vi "state_machine.vi"() -> ()   [LabVIEW 2023]
uses:
  typedefs/state_machine_types.ctl
panel:
  out "State":string
  in  "Up State":bool
  in  "Down State":bool
  in  "Stop Button":bool
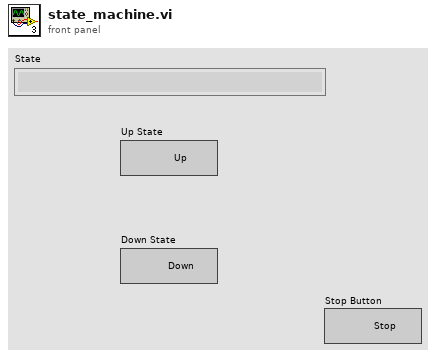
[diagram p1: front panel]
types:
  T1 = typedef "state_machine_types.ctl" = enum16{"Init", "Error", "Idle", "Down", "Up", "Next", "Previous", "Stop", ""}
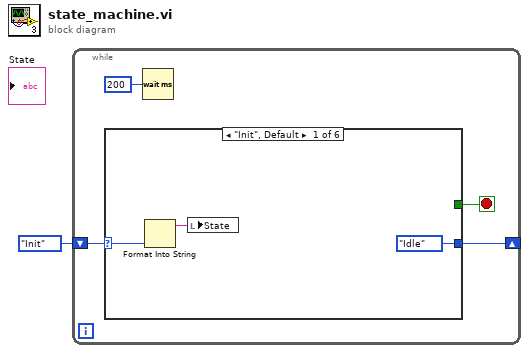
[diagram p0: block diagram]
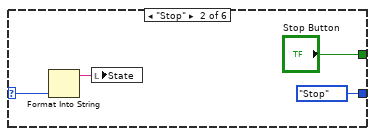
[diagram p2: hidden frame]
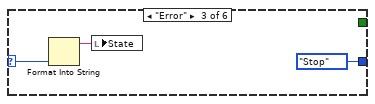
[diagram p3: hidden frame]
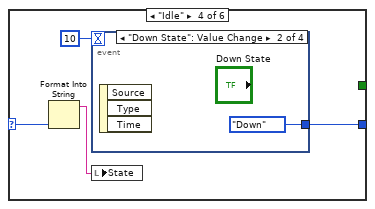
[diagram p4: hidden frame]
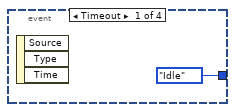
[diagram p5: hidden frame]
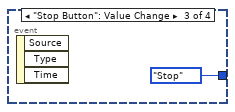
[diagram p6: hidden frame]
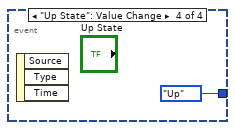
[diagram p7: hidden frame]
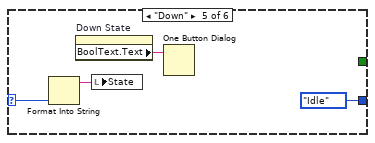
[diagram p8: hidden frame]
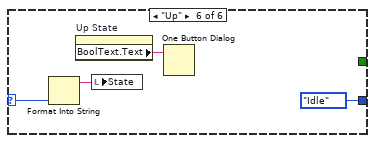
[diagram p9: hidden frame]
diagram:
  n1 = while {
    shift-right: [w4] -> _
    shift-left: state_machine_types."Init" -> [w2]
    stop <- w3 stop-if-true
    n2 = case shown="\"Init\", Default" w2 {
      selector: w2 -> [w7 w10 w14 w18 w24 w28]
      tunnel: [state_machine_types."Idle" state_machine_types."Stop" state_machine_types."Stop" w16 state_machine_types."Idle" state_machine_types."Idle"] -> w4
      tunnel: [_ "Stop Button" _ _ _ _] -> w3
      frame "Init", Default {
        n3 = Format Into String(w7) -> (resulting string=w6:string)  [unwired: 3 in, 1 out]
        n4 = local write "State"(w6) -> ()
      }
      frame "Stop" {
        n5 = Format Into String(w10) -> (resulting string=w9:string)  [unwired: 3 in, 1 out]
        n6 = local write "State"(w9) -> ()
      }
      frame "Error" {
        n7 = Format Into String(w14) -> (resulting string=w13:string)  [unwired: 3 in, 1 out]
        n8 = local write "State"(w13) -> ()
      }
      frame "Idle" {
        n9 = Format Into String(w18) -> (resulting string=w17:string)  [unwired: 3 in, 1 out]
        n10 = event shown="[1] \"Down State\": Value Change" {
          selector: _ -> [_ _ _ _]
          dyn-events: _ -> [_ _ _ _]
          timeout: 10 -> [_ _ _ _]
          tunnel: [state_machine_types."Idle" state_machine_types."Down" state_machine_types."Stop" state_machine_types."Up"] -> w16
          event Timeout {
            n11 = event-data() -> ()  [unwired: 1 in, 3 out]
          }
          event "Down State": Value Change {
            n12 = event-data() -> ()  [unwired: 1 in, 3 out]
          }
          event "Stop Button": Value Change {
            n13 = event-data() -> ()  [unwired: 1 in, 3 out]
          }
          event "Up State": Value Change {
            n14 = event-data() -> ()  [unwired: 1 in, 3 out]
          }
        }
        n15 = local write "State"(w17) -> ()
      }
      frame "Down" {
        n16 = Format Into String(w24) -> (resulting string=w25:string)  [unwired: 3 in, 1 out]
        n17 = property on="Down State" class="Bool"() -> ("BoolText.Text"=w27:string)  [unwired: 2 in, 2 out]
        n18 = local write "State"(w25) -> ()
        n19 = One Button Dialog(message=w27) -> ()  [unwired: 1 in, 1 out]
      }
      frame "Up" {
        n20 = Format Into String(w28) -> (resulting string=w29:string)  [unwired: 3 in, 1 out]
        n21 = property on="Up State" class="Bool"() -> ("BoolText.Text"=w31:string)  [unwired: 2 in, 2 out]
        n22 = local write "State"(w29) -> ()
        n23 = One Button Dialog(message=w31) -> ()  [unwired: 1 in, 1 out]
      }
    }
    n24 = Wait (ms)(milliseconds to wait=u32 200) -> ()  [unwired: 1 out]
  }
